vi "Main.vi"() -> ()   [LabVIEW 2023]
uses:
  States.ctl
  <vilib>/measure/NI_MAPro.lvlib
  <vilib>/measure/matone.llb/Extract Single Tone Information 1 Chan.vi
  <vilib>/DAQmx/read.llb/DAQmx Read (Analog 1D Wfm NChan NSamp).vi
  <vilib>/Waveform/WDTFileIO.llb/Write Waveforms to File (1D).vi
  Timing Params.ctl
  Channels.ctl
  Channel_choiche.ctl
panel:
  in  "Save waveform":bool
  in  "Save A":bool
  in  "Save Phase":bool
  in  "Channel 2":T1 items=["Vin", "Woofer", "Tweeter", "Midrange"]
  in  "Clear F":bool
  out "Phase analysis":cluster{"X":dbl, "Y":dbl}[](graph)
  in  "DAQ Parameters":T2={"Trigger Level"=0.0, "Sample Rate"=10000.0, "N Samples"=1000.0, "Trigger Slope"=10171, "Enable"=FALSE} {"Trigger Slope" items=["Falling"=10171, "Rising"=10280]; "Trigger Level" scale=-10.0..10.0}
  in  "Stop":bool
  in  "Channels":T3
  out "Data":waveform(dbl)[](graph)
  in  "Clear A":bool
  out "Freq Analysis":cluster{"X":dbl, "Y":dbl}[](graph)
  in  "Analizza F":bool
  in  "Channel":T1 items=["Vin", "Woofer", "Tweeter", "Midrange"]
  in  "DAQ":bool
  in  "Analizza A":bool
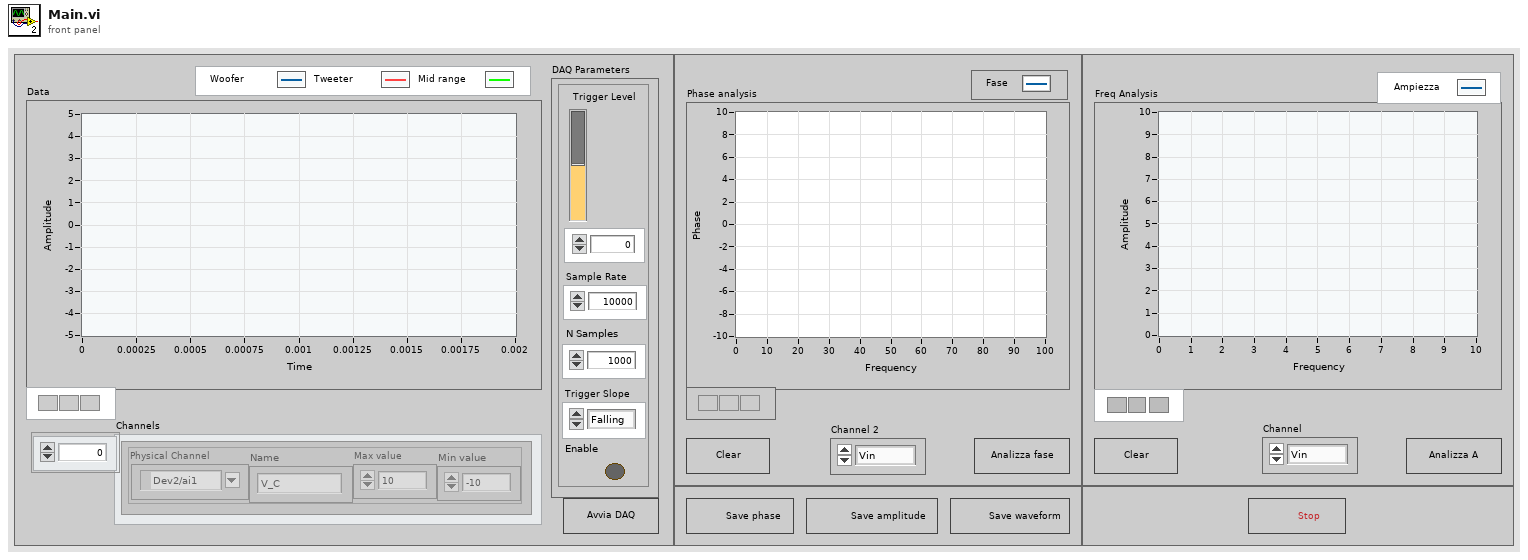
[diagram p1: front panel]
types:
  T1 = typedef "Channel_choiche.ctl" = i16
  T2 = typedef "Timing Params.ctl" = cluster{"Trigger Level":dbl, "Sample Rate":dbl, "N Samples":dbl, "Trigger Slope":u16, "Enable":bool}
  T3 = typedef "Channels.ctl" = cluster{"Physical Channel":tag, "Name":string, "Max value":dbl, "Min value":dbl}[]
  T4 = typedef "States.ctl" = enum16{"Idle", "Acquire", "Fit", "Stop", "Save"}
  T5 = cluster{"detected frequency":dbl, "detected amplitude":dbl}[]
  T6 = cluster{"detected frequency":dbl, "detected phase (deg)":dbl}[]
  T7 = cluster{"detected frequency":dbl, "detected amplitude":dbl}
  T8 = cluster{"detected frequency":dbl, "detected phase (deg)":dbl}
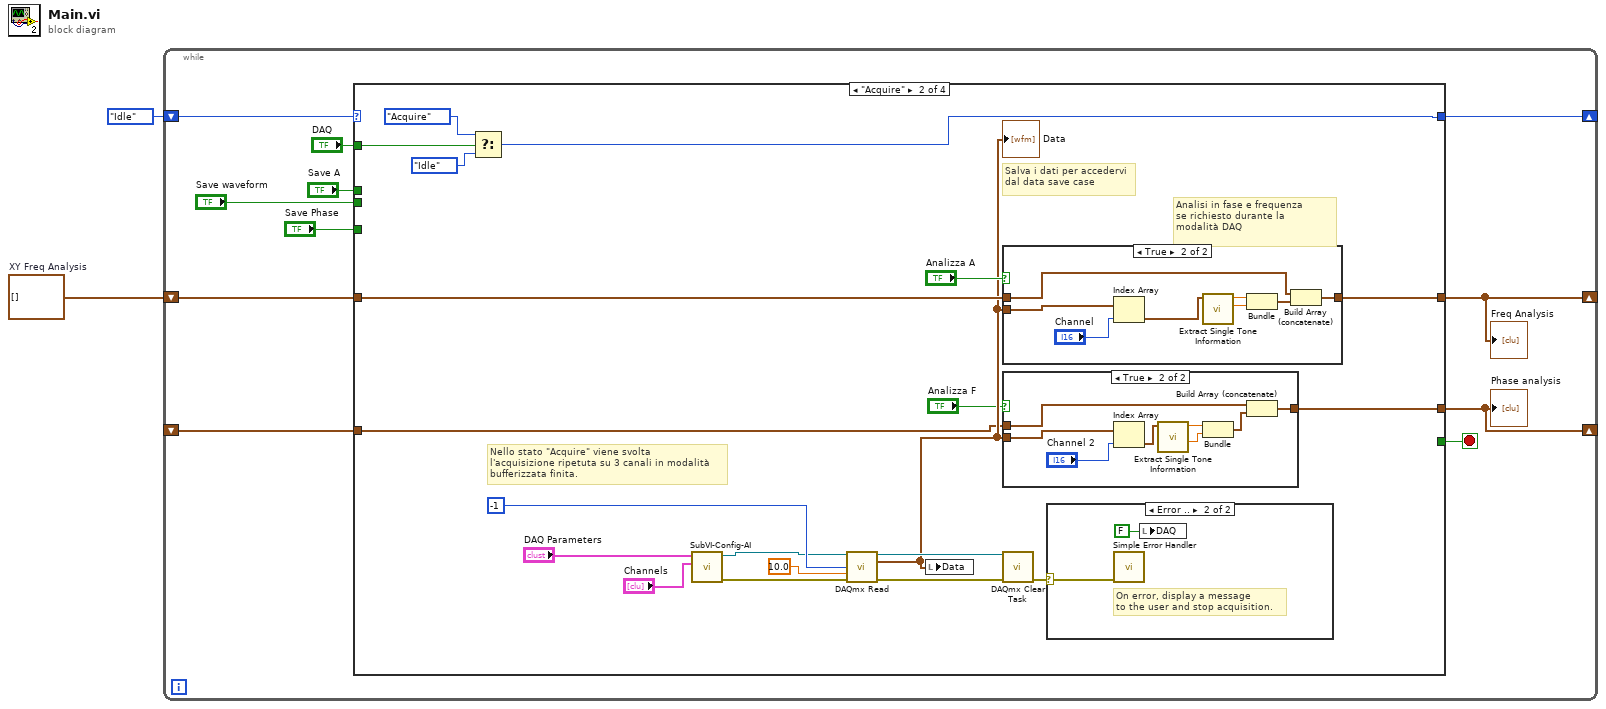
[diagram p0: block diagram]
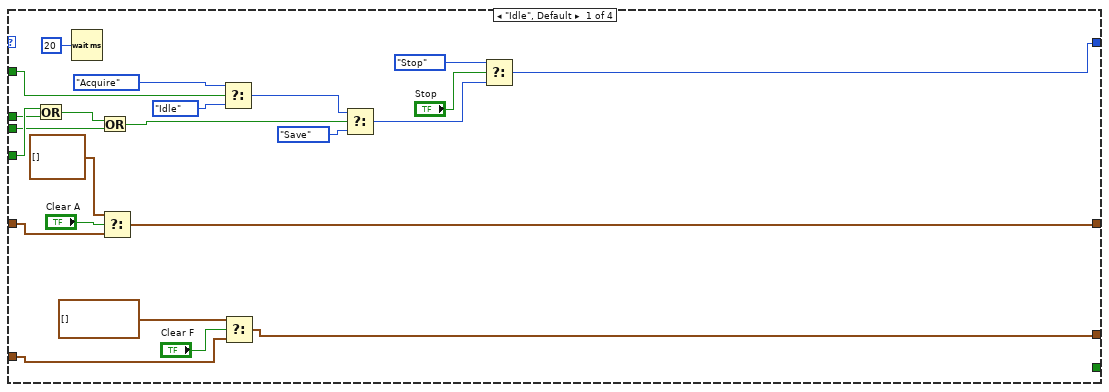
[diagram p2: hidden frame]
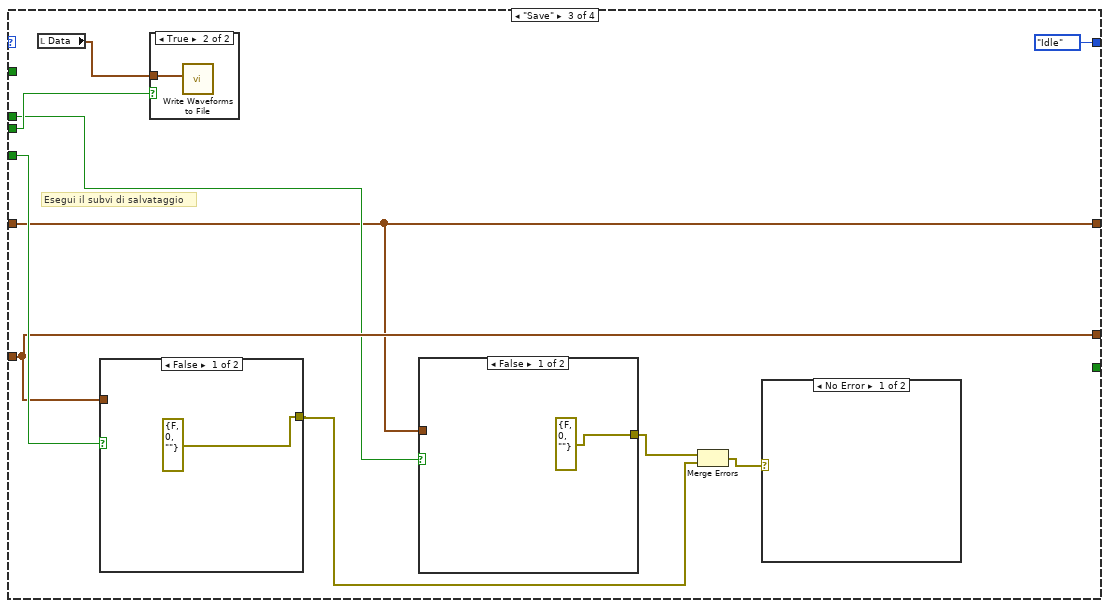
[diagram p6: hidden frame]
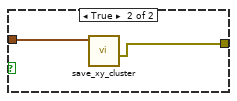
[diagram p8: hidden frame]
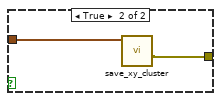
[diagram p10: hidden frame]
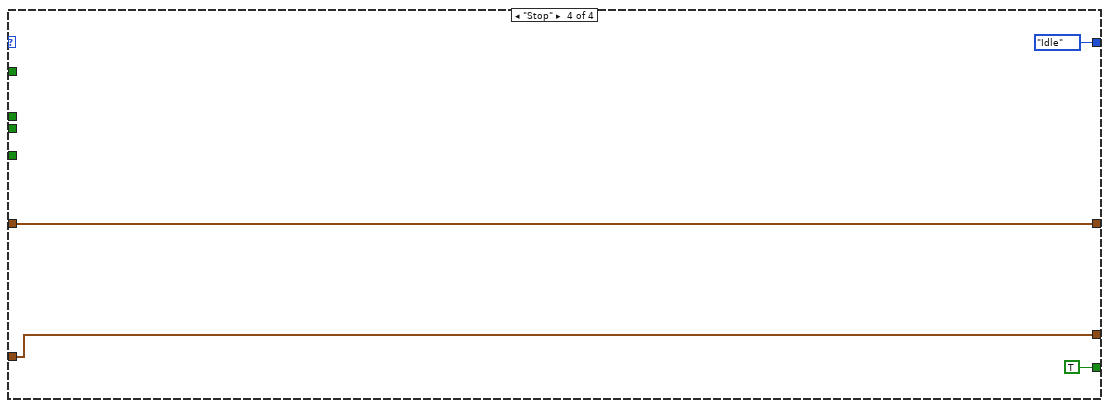
[diagram p11: hidden frame]
diagram:
  w2 = cluster{dbl, dbl}[] []  # XY Freq Analysis
  n1 = while {
    shift-right: [w10] -> _
    shift-left: w2 -> [w8]
    shift-right: [w11] -> _
    shift-left: States."Idle" ("Enum") -> [w13]
    shift-right: [w6] -> _
    shift-left: _ -> [w7]
    stop <- w9 stop-if-true
    n2 = case shown="\"Acquire\"" w13 {
      tunnel: "DAQ" -> [w34 w40 _ _]
      tunnel: w8 -> [w35 w46 w80 w97]
      tunnel: [w32 w37 States."Idle" ("Enum") States."Idle" ("Enum")] -> w11
      tunnel: [w29 w50 w80 w97] -> w10
      tunnel: [_ _ _ TRUE] -> w9
      tunnel: "Save waveform" -> [w20 _ w83 _]
      tunnel: w7 -> [w17 w42 w84 w94]
      tunnel: [w16 w41 w84 w94] -> w6
      tunnel: "Save Phase" -> [w22 _ w85 _]
      tunnel: "Save A" -> [w21 _ w81 _]
      frame "Idle", Default {
        n3 = Or(x=w22, y=w21) -> (x .or. y?=w19:bool)
        n4 = Wait (ms)(milliseconds to wait=u32 20) -> ()  [unwired: 1 out]
        n5 = Or(x=w19, y=w20) -> (x .or. y?=w18:bool)
        n6 = Select(t=cluster{dbl, dbl}[] [], s="Clear A", f=w35) -> (s? t:f=w29:T5)
        n7 = Select(t=States."Acquire" ("Enum"), s=w34, f=States."Idle" ("Enum")) -> (s? t:f=w28:T4)
        n8 = Select(t=cluster{dbl, dbl}[] [] ("Array"), s="Clear F", f=w17) -> (s? t:f=w16:T6)
        n9 = Select(t=w28, s=w18, f=States."Save" ("Enum")) -> (s? t:f=w27:T4)
        n10 = Select(t=States."Stop" ("Enum"), s="Stop", f=w27) -> (s? t:f=w32:T4)
      }
      frame "Acquire" {
        # "Analisi in fase e frequenza\nse richiesto durante la\nmodalità DAQ"
        # "Salva i dati per accedervi\ndal data save case"
        # "Nello stato \"Acquire\" viene svolta\nl'acquisizione ripetuta su 3 canali in modalità\nbufferizzata finita."
        n11 = Select(t=States."Acquire", s=w40, f=States."Idle" ("Enum")) -> (s? t:f=w37:T4)
        n12 = call "SubVI-Config-AI.vi"("Channels"="Channels", "Timing Params"="DAQ Parameters") -> ("error out"=w48:errorcluster, "Refnum out"=w49:refnum<k21>)  [unwired: 8 in]
        n13 = call-poly <vilib>:"DAQmx Read.vi"("task/channels in"=w49, "number of samples per channel"=-1, "timeout"=10.0, "error in"=w48) -> ("task out"=w54:refnum<k21>, "data"=w44:waveform(dbl)[], "error out"=w53:errorcluster)  [unwired: 9 in]
        "Data" <- w44
        n14 = local write "Data"(w44) -> ()
        n15 = case shown="True" "Analizza A" {
          tunnel: w44 -> [_ w74]
          tunnel: [w68 w75] -> w50
          tunnel: w46 -> [w68 w76]
          frame False {
          }
          frame True {
            n16 = Index Array "Index Array"(array=w74, index="Channel") -> (element=w72:waveform(dbl))
            n17 = call-poly <vilib>:"Extract Single Tone Information.vi"("time signal in"=w72) -> ("detected amplitude"=w70:dbl, "detected frequency"=w71:dbl)  [unwired: 5 in, 4 out]
            n18 = Bundle("detected frequency"=w71, "detected amplitude"=w70) -> (w69:T7)  [unwired: 1 in]
            n19 = Build Array (concatenate)(w76, w69) -> (w75:T5)
          }
        }
        n20 = case shown="True" "Analizza F" {
          tunnel: w44 -> [_ w64]
          tunnel: w42 -> [w57 w65]
          tunnel: [w57 w60] -> w41
          frame False {
          }
          frame True {
            n21 = Index Array(array=w64, index="Channel 2") -> (element=w63:waveform(dbl))
            n22 = call-poly <vilib>:"Extract Single Tone Information.vi"("time signal in"=w63) -> ("detected phase (deg)"=w61:dbl, "detected frequency"=w62:dbl)  [unwired: 5 in, 4 out]
            n23 = Bundle("detected frequency"=w62, "detected phase (deg)"=w61) -> (w58:T8)  [unwired: 1 in]
            n24 = Build Array (concatenate)(w65, w58) -> (w60:T6)
          }
        }
        n25 = call <vilib>:"DAQmx Clear Task.vi"("task in"=w54, "error in"=w53) -> ("error out"=w51:errorcluster)  [unwired: 13 in]
        n26 = case shown="Error .." w51 {
          selector: w51 -> [_ w67]
          frame No Error {
          }
          frame Error {
            # "On error, display a message\nto the user and stop acquisition."
            n27 = call <vilib>:"Simple Error Handler.vi"("error in (no error)"=w67) -> ()  [unwired: 4 in, 5 out]
            n28 = local write "DAQ"(FALSE ("DAQ")) -> ()
          }
        }
      }
      frame "Save" {
        # "Esegui il subvi di salvataggio"
        n29 = local read "Data"() -> (w82:waveform(dbl)[])
        n30 = case shown="False" w85 {
          tunnel: w84 -> [_ w93]
          tunnel: [errorcluster {"status"=FALSE, "code"=0, "source"=""} ("error in (no error)") w92] -> w78
          frame False {
          }
          frame True {
            n31 = call "save_xy_cluster.vi"("Array"=w93) -> ("error out"=w92:errorcluster)  [unwired: 10 in]
          }
        }
        n32 = case shown="True" w83 {
          tunnel: w82 -> [_ w90]
          frame False {
          }
          frame True {
            n33 = call-poly <vilib>:"Write Waveforms to File.vi"("waveform array"=w90) -> ()  [unwired: 9 in, 2 out]
          }
        }
        n34 = case shown="False" w81 {
          tunnel: w80 -> [_ w89]
          tunnel: [errorcluster {"status"=FALSE, "code"=0, "source"=""} ("error in (no error)") w88] -> w79
          frame False {
          }
          frame True {
            n35 = call "save_xy_cluster.vi"("Array"=w89) -> ("error out"=w88:errorcluster)  [unwired: 10 in]
          }
        }
        n36 = Merge Errors(w79, w78) -> (w77:errorcluster)
        n37 = case shown="No Error" w77 {
          frame No Error {
          }
          frame Error {
          }
        }
      }
      frame "Stop" {
      }
    }
    "Freq Analysis" <- w10
    "Phase analysis" <- w6
  }
